vi "AddItemsToGraph.vi"(0 "GraphIn":refnum<class "Graph.lvclass">, 1 "graphics":refnum<class "Graphics.lvclass">, 2 "grid":refnum<class "Grid.lvclass">, 3 "ClassNodes":T5(array[cluster]) {"Point"."y" format="%.2f"; "Point"."x" format="%.2f"}, 4 "NoteNodes":T4(array[cluster]) {"Point"."y" format="%.2f"; "Point"."x" format="%.2f"}, 5 "error in (no error)":errorcluster, 7 "Links":T1[](array[typedef]), 9 "DoAContainCheck":bool, 11 "ClassNodesAtt/MethodIDs":cluster{string[], string[]}[](array[cluster]), 13 "NodeIndexiesToOnlyUpdate":i32[](array[numeric])) -> (14 "GraphOut":refnum<class "Graph.lvclass">, 16 "NodesCreated/Modified":refnum<class "AbstractNode.lvclass">[](array[class]), 19 "error out":errorcluster)   [LabVIEW 2020, in "Graph.lvclass"]
uses:
  <resource>/Framework/Providers/Open_GDS/UML/Graph_class/Graph.lvclass
  <resource>/Framework/Providers/Open_GDS/UML/Graphics_class/Graphics.lvclass
  <resource>/Framework/Providers/Open_GDS/UML/Grid_class/Grid.lvclass
  <resource>/Framework/Providers/Open_GDS/UML/General/Point/Point Point2D.ctl
  <resource>/Framework/Providers/Open_GDS/UML/Graph_class/AddItemsToGraph_Edges.ctl
  <resource>/Framework/Providers/Open_GDS/UML/DesignPattern/SubVIs/DesignPatterns_LinkType.ctl
  <resource>/Framework/Providers/Open_GDS/UML/AbstractNode_class/AbstractNode.lvclass
  <resource>/Framework/Providers/Open_GDS/UML/ClassNode_class/ClassNode.lvclass
  C:/Program Files (x86)/National Instruments/LabVIEW 2020/resource/Framework/Providers/Open_GDS/UML/AbstractNode_class/AbstractNode.lvclass
  <resource>/Framework/Providers/Open_GDS/UML/AbstractEdge_class/AbstractEdge.lvclass
  <resource>/Framework/Providers/Open_GDS/UML/ClassNode_class/ExternalSetTypes.ctl
  <resource>/Framework/Providers/Open_GDS/UML/MultiLineString_class/JustificationType.ctl
  <resource>/Framework/Providers/Open_GDS/UML/ClassRelationshipEdge_class/ExternaSetParamType.ctl
  <resource>/Framework/Providers/Open_GDS/UML/BentStyle_class/BentStyleType.ctl
  <resource>/Framework/Providers/Open_GDS/UML/ArrowHead_class/ArrowHeadType.ctl
  <resource>/Framework/Providers/Open_GDS/UML/LineStyle_class/LineStyleType.ctl
  <resource>/Framework/Providers/Open_GDS/UML/InterfaceNode_class/InterfaceNode.lvclass
  C:/Program Files (x86)/National Instruments/LabVIEW 2020/resource/Framework/Providers/Open_GDS/UML/ClassNode_class/ClassNode.lvclass
  <resource>/Framework/Providers/Open_GDS/UML/NoteNode_class/NoteNode.lvclass
  <resource>/Framework/Providers/Open_GDS/UML/ClassRelationshipEdge_class/ClassRelationshipEdge.lvclass
  C:/Program Files (x86)/National Instruments/LabVIEW 2020/resource/Framework/Providers/Open_GDS/UML/AbstractEdge_class/AbstractEdge.lvclass
  <resource>/Framework/Providers/Open_GDS/UML/NoteEdge_class/NoteEdge.lvclass
  <resource>/Framework/Providers/Open_GDS/UML/LineStyle_class/LineStyle.lvclass
  <resource>/Framework/Providers/Open_GDS/UML/MultiLineString_class/MultiLineString.lvclass
  <resource>/Framework/Providers/Open_GDS/UML/ArrowHead_class/ArrowHead.lvclass
  <resource>/Framework/Providers/Open_GDS/UML/BentStyle_class/BentStyle.lvclass
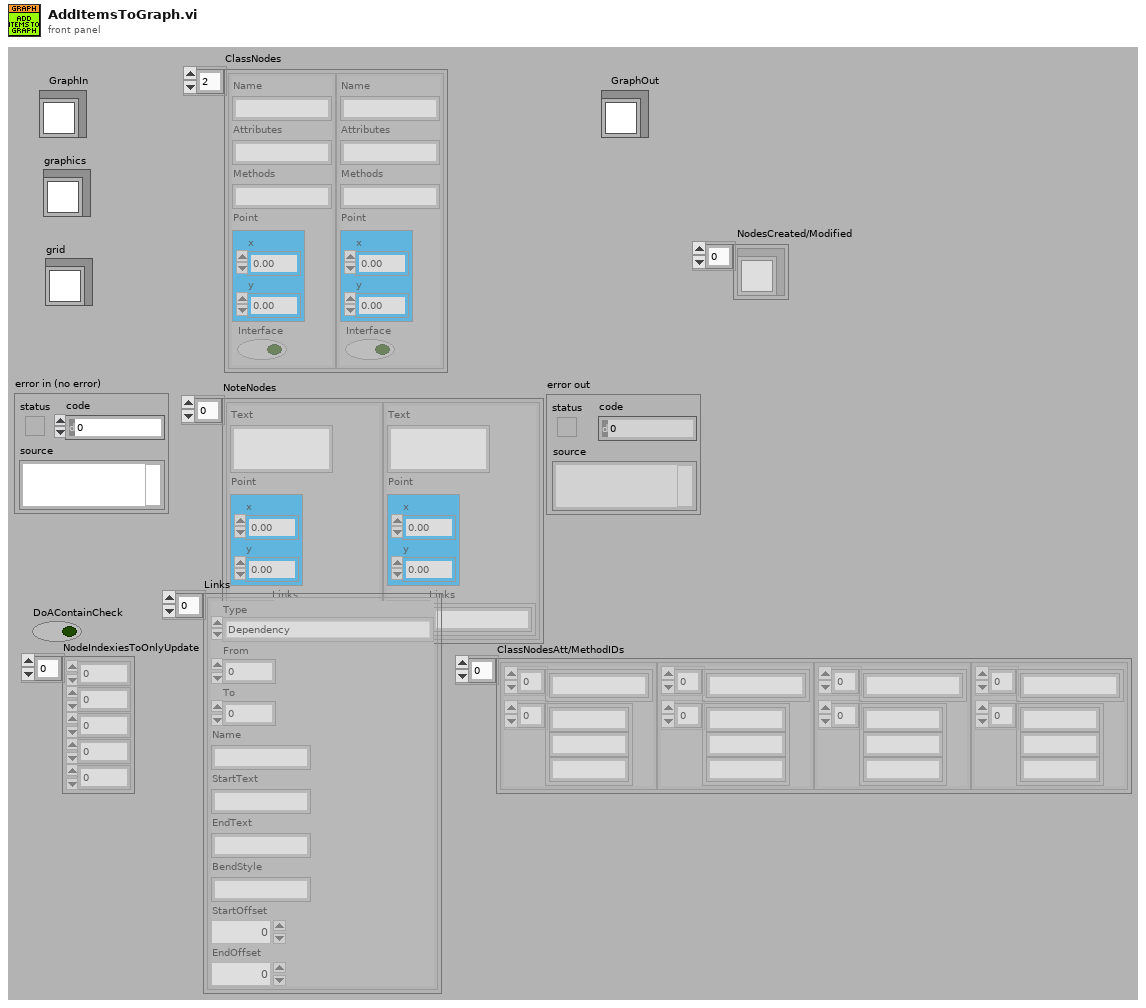
[diagram p1: front panel]
types:
  T1 = typedef "Graph.lvclass/AddItemsToGraph_Edges.ctl" = cluster{"Type":T2, "From":i32, "To":i32, "Name":string, "StartText":string, "EndText":string, "BendStyle":string, "StartOffset":i32, "EndOffset":i32}
  T2 = typedef "DesignPatterns_LinkType.ctl" = enum16{"Dependency", "Inheritance", "Interface", "Association", "Aggregation", "CompositeAggregation"}
  T3 = typedef "Point Point2D.ctl" = cluster{"x":dbl, "y":dbl}
  T4 = cluster{"Text":string, "Point":T3, "Links":string[]}[]
  T5 = cluster{"Name":string, "Attributes":string, "Methods":string, "Point":T3, "Interface":bool}[]
  T6 = cluster{"Text":string, "Cancelled":bool, "Classes":refnum<class "ClassNode.lvclass">[], "Edges":refnum<class "AbstractEdge.lvclass">[], "Notes":refnum<class "AbstractNode.lvclass">[], "NoteLinks":cluster{cluster{"reference out":refnum<class "ClassNode.lvclass">, "RightPoint":T3}[]}[], "ClassNodes":cluster{"Name":string, "Attributes":string, "Methods":string, "Point":T3, "Interface":bool}[], "Offset":T3, "nodes":refnum<class "AbstractNode.lvclass">[]}
  T7 = typedef "ClassNode.lvclass/ExternalSetTypes.ctl" = enum16{"Name", "Attributes", "Methods", "Position", "ShowMethods", "ShowAttributes", "ClassPath"}
  T8 = cluster{"reference out":refnum<class "ClassNode.lvclass">, "RightPoint":T3}[]
  T9 = typedef "MultiLineString.lvclass/JustificationType.ctl" = enum16{"LEFT", "CENTER", "RIGHT"}
  T10 = typedef "ClassRelationshipEdge.lvclass/ExternaSetParamType.ctl" = enum16{"StartLabel", "MidLabel", "EndLabel", "StartNode", "EndNode", "BendType", "StartArrow", "EndArrow", "StartOffset", "EndOffset"}
  T11 = typedef "BentStyle.lvclass/BentStyleType.ctl" = enum16{"STRAIGHT", "HV", "VH", "HVH", "VHV", "ARC"}
  T12 = typedef "ArrowHead.lvclass/ArrowHeadType.ctl" = enum16{"NONE", "TRIANGLE", "BLACK_TRIANGLE", "V", "HALF_V", "DIAMOND", "BLACK_DIAMOND"}
  T13 = typedef "LineStyle.lvclass/LineStyleType.ctl" = enum16{"SOLID", "DOTTED"}
  T14 = typedef "Rectangle Rectangle2D.ctl" = cluster{"x":dbl, "y":dbl, "width":dbl, "height":dbl}
  T15 = cluster{"Name":string, "Attributes":string, "Methods":string, "Point":T3, "Interface":bool}
  T16 = cluster{"reference out":refnum<class "ClassNode.lvclass">, "RightPoint":T3}
  T17 = cluster{"reference out":refnum<class "ClassNode.lvclass">, "UpperRightPoint":T3}
  T18 = cluster{"reference out":refnum<class "ClassNode.lvclass">, "UpperRightPoint":T3}[]
  T19 = cluster{cluster{"reference out":refnum<class "ClassNode.lvclass">, "RightPoint":T3}[]}
  T20 = cluster{cluster{"reference out":refnum<class "ClassNode.lvclass">, "RightPoint":T3}[]}[]
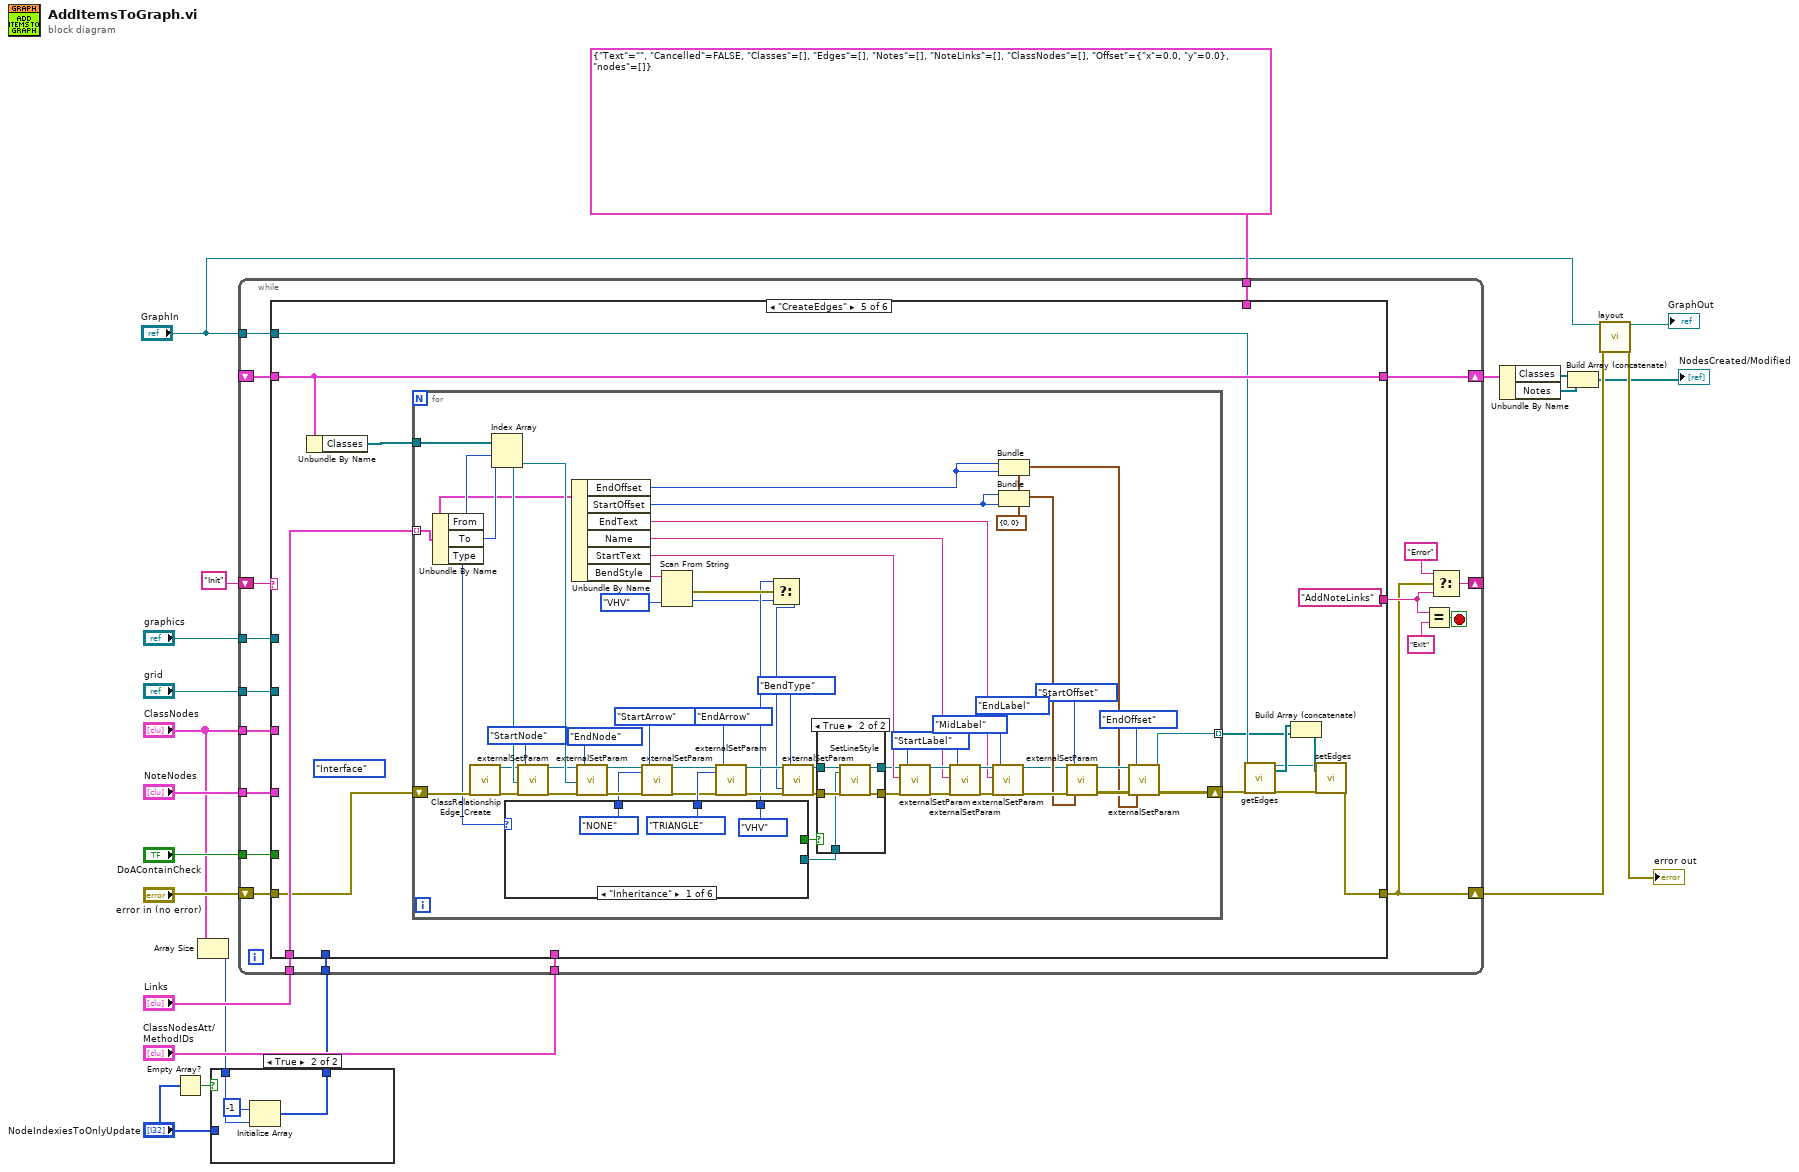
[diagram p0: block diagram]
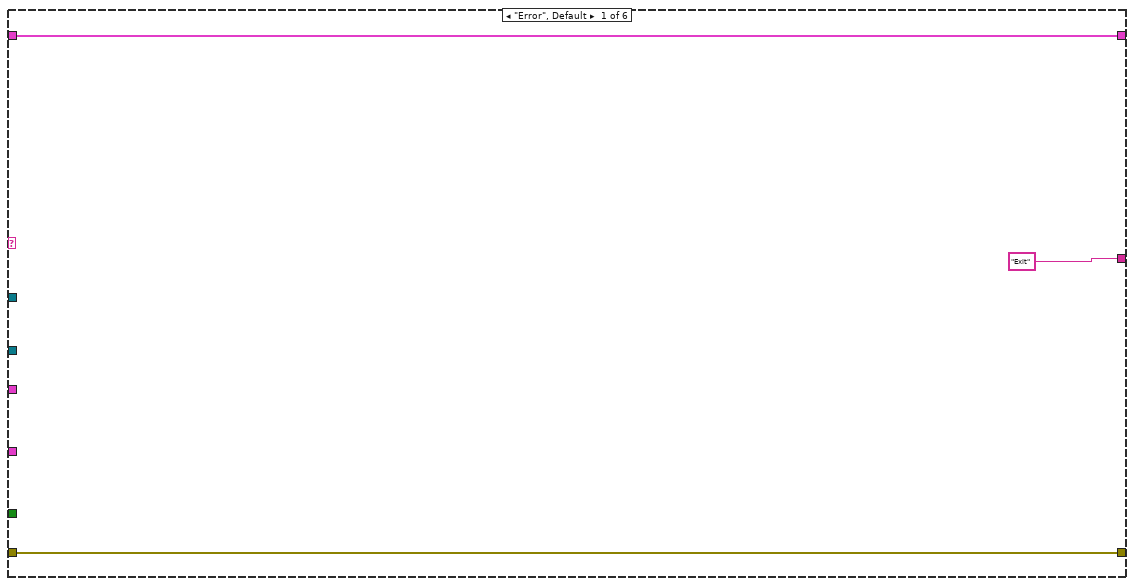
[diagram p3: hidden frame]
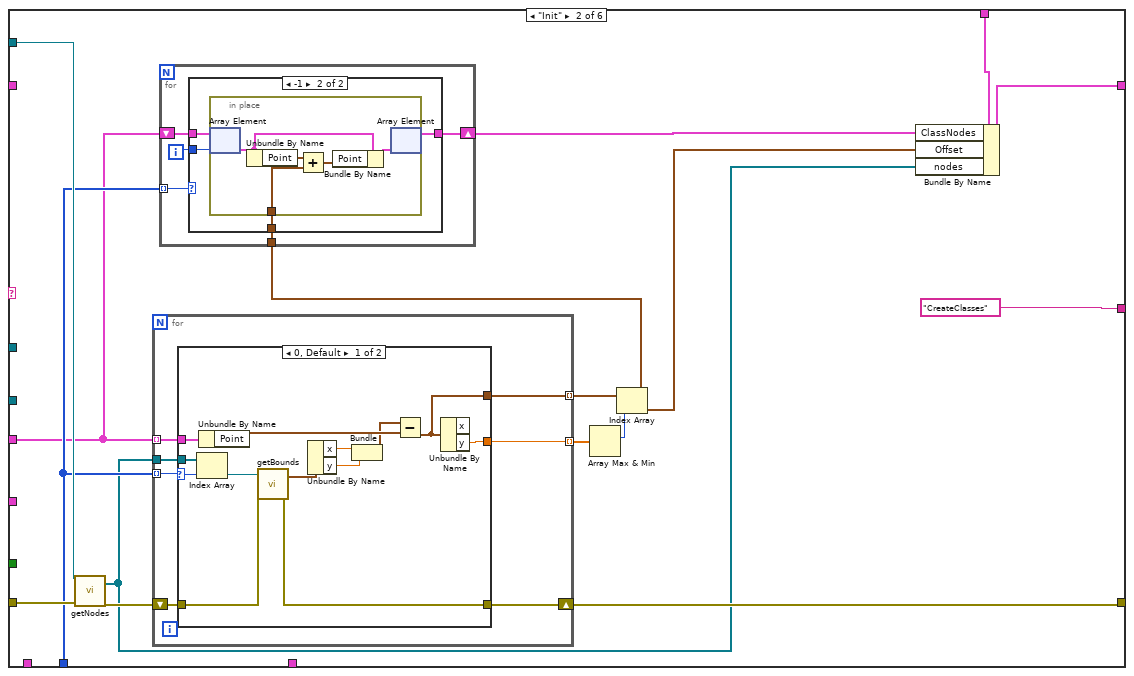
[diagram p4: hidden frame]
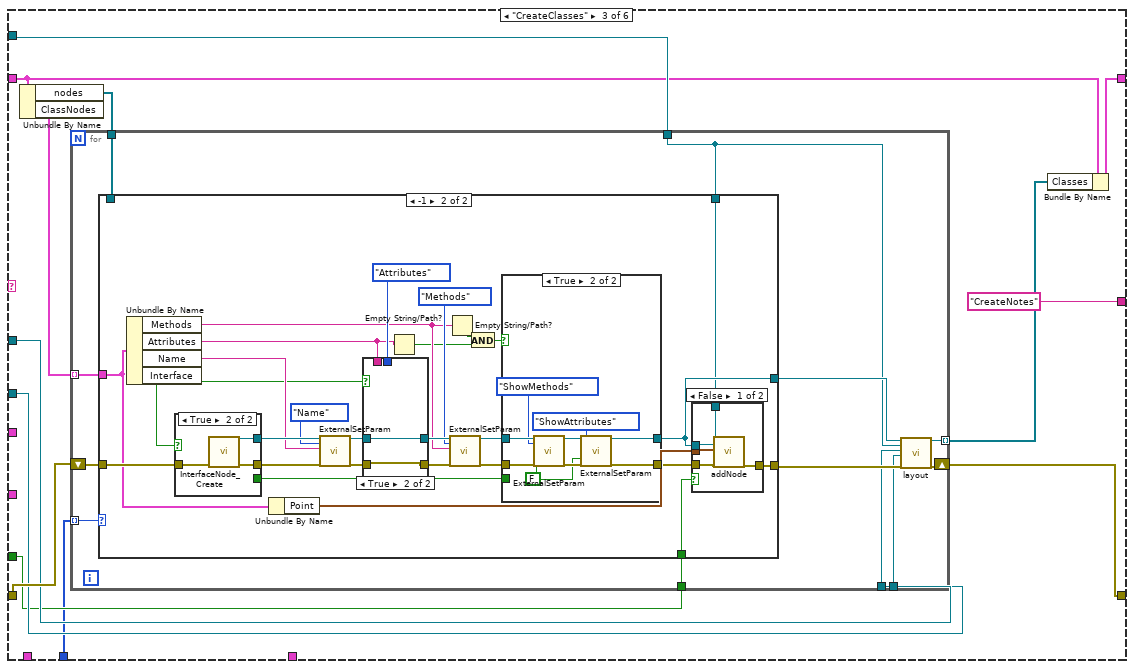
[diagram p7: hidden frame]
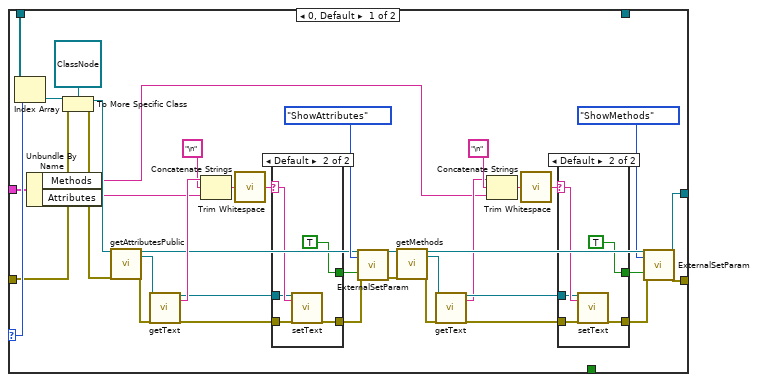
[diagram p8: hidden frame]
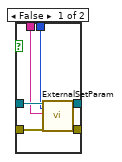
[diagram p11: hidden frame]
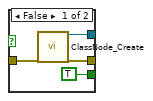
[diagram p12: hidden frame]
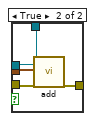
[diagram p14: hidden frame]
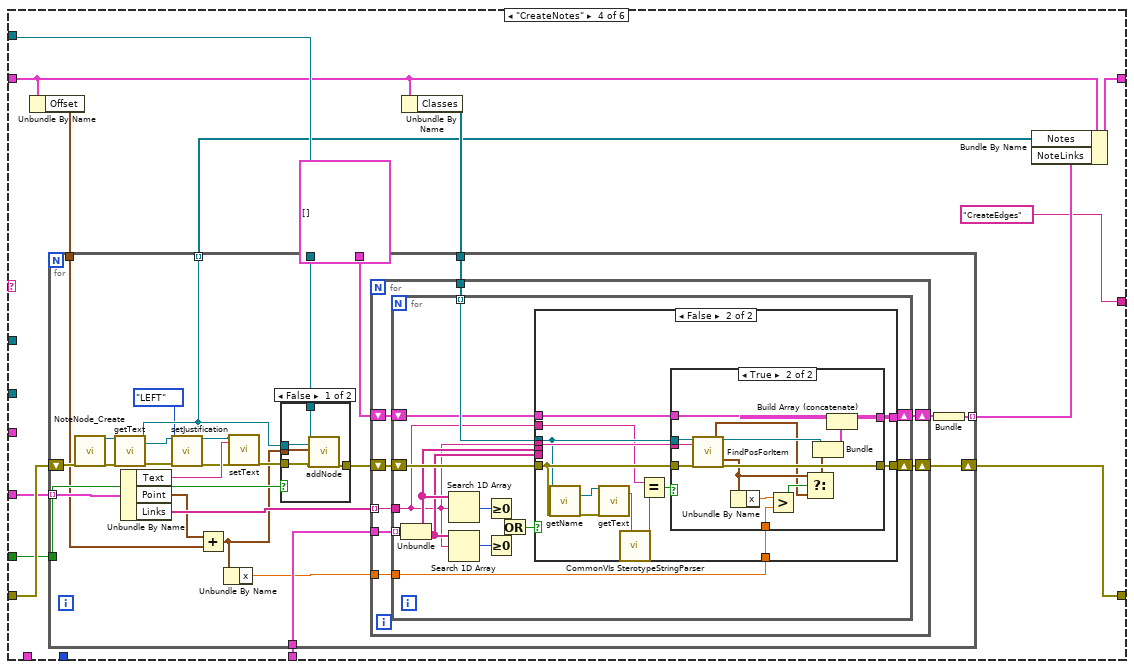
[diagram p15: hidden frame]
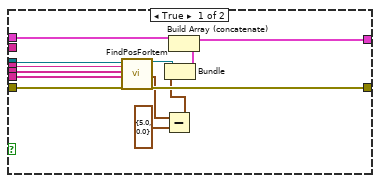
[diagram p16: hidden frame]
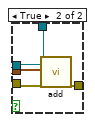
[diagram p18: hidden frame]
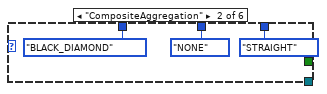
[diagram p20: hidden frame]
diagram:
  n1 = Empty Array?(array="NodeIndexiesToOnlyUpdate") -> (empty?=w8:bool)
  n2 = Array Size(array="ClassNodes") -> (size(s)=w5:i32)
  n3 = case shown="True" w8 {
    tunnel: "NodeIndexiesToOnlyUpdate" -> [w23 _]
    tunnel: w5 -> [_ w25]
    tunnel: [w23 w24] -> w4
    frame False {
    }
    frame True {
      n4 = Initialize Array(-1, w25) -> (w24:i32[])
    }
  }
  n5 = while {
    shift-right: [w39] -> w13
    shift-left: "error in (no error)" -> [w46]
    shift-right: [w44] -> _
    shift-left: "Init" -> [w45]
    shift-right: [w38] -> w22
    shift-left: _ -> [w37]
    tunnel: "GraphIn" -> [w36]
    tunnel: "graphics" -> [w35]
    tunnel: "grid" -> [w34]
    tunnel: T6 {"Text"="", "Cancelled"=FALSE, "Classes"=[], "Edges"=[], "Notes"=[], "NoteLinks"=[], "ClassNodes"=[], "Offset"={"x"=0.0, "y"=0.0}, "nodes"=[]} -> [w33]
    tunnel: "ClassNodes" -> [w27]
    tunnel: "NoteNodes" -> [w32]
    tunnel: "DoAContainCheck" -> [w31]
    tunnel: "Links" -> [w30]
    tunnel: "ClassNodesAtt/MethodIDs" -> [w29]
    tunnel: w4 -> [w28]
    stop <- w43 stop-if-true
    n6 = case shown="\"CreateEdges\"" w45 {
      tunnel: w46 -> [w49 w61 w111 w251 w363 w464]
      tunnel: [w49 w58 w110 w250 w362 w462] -> w39
      tunnel: ["Exit" "CreateClasses" "CreateNotes" "CreateEdges" "AddNoteLinks" "Exit"] -> w40
      tunnel: [w47 w63 w109 w245 w360 w458] -> w38
      tunnel: w37 -> [w47 _ w105 w242 w360 w459]
      tunnel: w36 -> [_ w60 w112 w252 w355 w463]
      tunnel: w35 -> [_ _ w107 _ _ _]
      tunnel: w34 -> [_ _ w106 _ _ _]
      tunnel: w33 -> [_ w62 _ _ _ _]
      tunnel: w32 -> [_ _ _ w249 _ _]
      tunnel: w31 -> [_ _ w103 w248 _ _]
      tunnel: w30 -> [_ _ _ _ w364 _]
      tunnel: w29 -> [_ _ _ w247 _ _]
      tunnel: w28 -> [_ w54 w102 _ _ _]
      tunnel: w27 -> [_ w52 _ _ _ _]
      frame "Error", Default {
      }
      frame "Init" {
        n7 = call-dynamic "getNodes.vi"("reference"=w60, "error in (no error)"=w61) -> ("nodes"=w50:refnum<class "AbstractNode.lvclass">[], "error out"=w59:errorcluster)  [unwired: 15 in, 1 out]
        n8 = for {
          tunnel: w50 -> [w86]
          tunnel: w54 -> [w83] mode=indexing
          shift-right: [w84] -> w58
          shift-left: w59 -> [w85]
          tunnel: w52 -> [w82] mode=indexing
          tunnel: [w81] -> w56 mode=indexing
          tunnel: [w80] -> w57 mode=indexing
          n9 = case shown="0, Default" w83 {
            selector: w83 -> [w95 _]
            tunnel: w86 -> [w99 _]
            tunnel: w85 -> [w97 w100]
            tunnel: [w96 w100] -> w84
            tunnel: w82 -> [w94 _]
            tunnel: [w88 _] -> w81
            tunnel: [w87 _] -> w80
            frame 0, Default {
              n10 = Index Array(array=w99, index=w95) -> (element=w98:refnum<class "AbstractNode.lvclass">)
              n11 = Unbundle By Name(w94) -> ("Point"=w90:T3)
              n12 = call-dynamic "getBounds.vi"("reference"=w98, "error in (no error)"=w97) -> ("bounds"=w93:T14, "error out"=w96:errorcluster)  [unwired: 15 in, 1 out]
              n13 = Unbundle By Name(w93) -> ("x"=w92:dbl, "y"=w91:dbl)
              n14 = Bundle("x"=w92, "y"=w91) -> (w89:cluster{"x":dbl, "y":dbl})  [unwired: 1 in]
              n15 = Subtract(x=w89, y=w90) -> (x-y=w88:T3)
              n16 = Unbundle By Name(w88) -> ("y"=w87:dbl)  [unwired: 1 out]
            }
            frame -1 {
            }
          }
        }
        n17 = Array Max & Min(array=w57) -> (max index (indices)=w55:i32)  [unwired: 3 out]
        n18 = Index Array(array=w56, index=w55) -> (element=w51:T3)
        n19 = for {
          tunnel: w54 -> [w69] mode=indexing
          tunnel: w51 -> [w67]
          shift-right: [w66] -> w53
          shift-left: w52 -> [w68]
          i -> [w65]
          n20 = case shown="-1" w69 {
            tunnel: w68 -> [w70 w73]
            tunnel: w67 -> [_ w74]
            tunnel: [w70 w72] -> w66
            tunnel: w65 -> [_ w71]
            frame 0, Default {
            }
            frame -1 {
              n21 = in-place {
                in-place-border: w74 -> [w77]
                n22 = in-place-array #1(w73, w71) -> (w76:T15)
                n23 = Unbundle By Name(w76) -> ("Point"=w79:T3)
                n24 = Add(x=w79, y=w77) -> (x+y=w78:T3)
                n25 = Bundle By Name(cluster=w76, "Point"=w78) -> (w75:T15)
                n26 = in-place-array #1(w75) -> (w72:T5)  [unwired: 1 out]
              }
            }
          }
        }
        n27 = Bundle By Name(cluster=w62, "ClassNodes"=w53, "Offset"=w51, "nodes"=w50) -> (w63:T6)
      }
      frame "CreateClasses" {
        n28 = Unbundle By Name(w105) -> ("nodes"=w101:refnum<class "AbstractNode.lvclass">[], "ClassNodes"=w104:T5)
        n29 = for {
          tunnel: w104 -> [w125] mode=indexing
          tunnel: w112 -> [w116]
          shift-right: [w121] -> w110
          shift-left: w111 -> [w124]
          tunnel: w103 -> [w123]
          tunnel: [w120] -> w108 mode=indexing
          tunnel: w107 -> [w119]
          tunnel: w106 -> [w118]
          tunnel: w102 -> [w114] mode=indexing
          tunnel: w101 -> [w115]
          n30 = case shown="-1" w114 {
            selector: w114 -> [w162 _]
            tunnel: w125 -> [w158 w178]
            tunnel: w124 -> [w160 w192]
            tunnel: w123 -> [_ w191]
            tunnel: [w127 w189] -> w122
            tunnel: [w126 w186] -> w117
            tunnel: w116 -> [_ w179]
            tunnel: w115 -> [w163 _]
            frame 0, Default {
              n31 = Index Array(array=w163, index=w162) -> (element=w161:refnum<class "AbstractNode.lvclass">)
              n32 = Unbundle By Name(w158) -> ("Methods"=w128:string, "Attributes"=w151:string)
              n33 = To More Specific Class(target class=refnum<class "ClassNode.lvclass"> refnum ("reference"), reference=w161, error in=w160) -> (specific class reference=w156:refnum<class "ClassNode.lvclass">, error out=w157:errorcluster)
              n34 = call <resource>:"getAttributesPublic.vi"("reference"=w156, "error in (no error)"=w157) -> ("reference out"=w144:refnum<class "ClassNode.lvclass">, "methods"=w154:refnum<class "MultiLineString.lvclass">, "error out"=w155:errorcluster)  [unwired: 15 in]
              n35 = call-dynamic "getText.vi"("reference"=w154, "error in (no error)"=w155) -> ("reference out"=w147:refnum<class "MultiLineString.lvclass">, "text"=w153:string, "error out"=w148:errorcluster)  [unwired: 15 in]
              n36 = Concatenate Strings(w153, "\n" ("string"), w151) -> (w150:string)
              n37 = call <vilib>:"Trim Whitespace.vi"("string"=w150) -> ("trimmed string"=w149:string)  [unwired: 1 in]
              n38 = case shown="Default" w149 {
                selector: w149 -> [_ w174]
                tunnel: w148 -> [w170 w175]
                tunnel: w147 -> [_ w173]
                tunnel: [w170 w172] -> w146
                tunnel: [_ TRUE] -> w143
                frame "" {
                }
                frame Default {
                  n39 = call-dynamic "setText.vi"("reference"=w173, "text"=w174, "error in (no error)"=w175) -> ("error out"=w172:errorcluster)  [unwired: 15 in, 1 out]
                }
              }
              n40 = call-dynamic "ExternalSetParam.vi"("reference"=w144, "setParameter"=ExternalSetTypes."ShowAttributes", "Boolean"=w143, "error in (no error)"=w146) -> ("reference out"=w130:refnum<class "ClassNode.lvclass">, "error out"=w129:errorcluster)  [unwired: 14 in]
              n41 = call <resource>:"getMethods.vi"("reference"=w130, "error in (no error)"=w129) -> ("reference out"=w141:refnum<class "ClassNode.lvclass">, "methods"=w132:refnum<class "MultiLineString.lvclass">, "error out"=w131:errorcluster)  [unwired: 15 in]
              n42 = call-dynamic "getText.vi"("reference"=w132, "error in (no error)"=w131) -> ("reference out"=w138:refnum<class "MultiLineString.lvclass">, "text"=w133:string, "error out"=w137:errorcluster)  [unwired: 15 in]
              n43 = Concatenate Strings(w133, "\n" ("string"), w128) -> (w135:string)
              n44 = call <vilib>:"Trim Whitespace.vi"("string"=w135) -> ("trimmed string"=w136:string)  [unwired: 1 in]
              n45 = case shown="Default" w136 {
                selector: w136 -> [_ w168]
                tunnel: w137 -> [w164 w169]
                tunnel: w138 -> [_ w167]
                tunnel: [w164 w166] -> w139
                tunnel: [_ TRUE] -> w142
                frame "" {
                }
                frame Default {
                  n46 = call-dynamic "setText.vi"("reference"=w167, "text"=w168, "error in (no error)"=w169) -> ("error out"=w166:errorcluster)  [unwired: 15 in, 1 out]
                }
              }
              n47 = call-dynamic "ExternalSetParam.vi"("reference"=w141, "setParameter"=ExternalSetTypes."ShowMethods", "Boolean"=w142, "error in (no error)"=w139) -> ("reference out"=w126:refnum<class "ClassNode.lvclass">, "error out"=w127:errorcluster)  [unwired: 14 in]
            }
            frame -1 {
              n48 = Unbundle By Name(w178) -> ("Methods"=w184:string, "Attributes"=w183:string, "Name"=w193:string, "Interface"=w177:bool)
              n49 = case shown="True" w177 {
                tunnel: [w214 w215] -> w202
                tunnel: [w213 w217] -> w201
                tunnel: w192 -> [w212 w216]
                tunnel: [TRUE ("Boolean") _] -> w176
                frame False {
                  n50 = call <resource>:"ClassNode_Create.vi"("error in (no error)"=w212) -> ("reference out"=w214:refnum<class "ClassNode.lvclass">, "error out"=w213:errorcluster)  [unwired: 1 in, 16 out]
                }
                frame True {
                  n51 = call <resource>:"InterfaceNode_Create.vi"("error in (no error)"=w216) -> ("reference out"=w215:refnum<class "InterfaceNode.lvclass">, "error out"=w217:errorcluster)  [unwired: 17 in]
                }
              }
              n52 = Unbundle By Name(w178) -> ("Point"=w190:T3)
              n53 = call-dynamic "ExternalSetParam.vi"("reference"=w202, "setParameter"=ExternalSetTypes."Name", "string"=w193, "error in (no error)"=w201) -> ("reference out"=w199:refnum<class "ClassNode.lvclass">, "error out"=w198:errorcluster)  [unwired: 14 in]
              n54 = case shown="True" w177 {
                tunnel: w199 -> [w208 w210]
                tunnel: w198 -> [w207 w209]
                tunnel: ExternalSetTypes."Attributes" ("setParameter") -> [w206 _]
                tunnel: [w205 w209] -> w196
                tunnel: [w204 w210] -> w195
                tunnel: w183 -> [w203 _]
                frame False {
                  n55 = call-dynamic "ExternalSetParam.vi"("reference"=w208, "setParameter"=w206, "string"=w203, "error in (no error)"=w207) -> ("reference out"=w204:refnum<class "ClassNode.lvclass">, "error out"=w205:errorcluster)  [unwired: 14 in]
                }
                frame True {
                }
              }
              n56 = Empty String/Path?(string/path=w183) -> (empty?=w181:bool)
              n57 = Empty String/Path?(string/path=w184) -> (empty?=w182:bool)
              n58 = call-dynamic "ExternalSetParam.vi"("reference"=w195, "setParameter"=ExternalSetTypes."Methods", "string"=w184, "error in (no error)"=w196) -> ("reference out"=w185:refnum<class "ClassNode.lvclass">, "error out"=w188:errorcluster)  [unwired: 14 in]
              n59 = And(x=w182, y=w181) -> (x .and. y?=w180:bool)
              n60 = case shown="True" w180 {
                tunnel: w188 -> [w218 w228]
                tunnel: [w218 w226] -> w187
                tunnel: [w219 w225] -> w186
                tunnel: w185 -> [w219 w223]
                tunnel: w176 -> [_ _]
                frame False {
                }
                frame True {
                  w220 = FALSE ("Boolean")
                  n61 = call-dynamic "ExternalSetParam.vi"("reference"=w223, "setParameter"=ExternalSetTypes."ShowMethods", "Boolean"=w220, "error in (no error)"=w228) -> ("reference out"=w224:refnum<class "ClassNode.lvclass">, "error out"=w227:errorcluster)  [unwired: 14 in]
                  n62 = call-dynamic "ExternalSetParam.vi"("reference"=w224, "setParameter"=ExternalSetTypes."ShowAttributes", "Boolean"=w220, "error in (no error)"=w227) -> ("reference out"=w225:refnum<class "ClassNode.lvclass">, "error out"=w226:errorcluster)  [unwired: 14 in]
                }
              }
              n63 = case shown="False" w191 {
                tunnel: w179 -> [w232 w238]
                tunnel: w190 -> [w233 w237]
                tunnel: [w229 w236] -> w189
                tunnel: w186 -> [w231 w235]
                tunnel: w187 -> [w230 w234]
                frame False {
                  n64 = call-dynamic "addNode.vi"("reference"=w232, "node"=w231, "point"=w233, "error in (no error)"=w230) -> ("error out"=w229:errorcluster)  [unwired: 14 in, 1 out]
                }
                frame True {
                  n65 = call-dynamic "add.vi"("reference"=w238, "node"=w235, "point"=w237, "error in (no error)"=w234) -> ("error out"=w236:errorcluster)  [unwired: 13 in, 2 out]
                }
              }
            }
          }
          n66 = call-dynamic "layout.vi"("reference"=w117, "graph"=w116, "graphics"=w119, "grid"=w118, "error in (no error)"=w122) -> ("reference out"=w120:refnum<class "ClassNode.lvclass">, "error out"=w121:errorcluster)  [unwired: 13 in]
        }
        n67 = Bundle By Name(cluster=w105, "Classes"=w108) -> (w109:T6)
      }
      frame "CreateNotes" {
        n68 = Unbundle By Name(w242) -> ("Offset"=w241:T3)
        n69 = Unbundle By Name(w242) -> ("Classes"=w246:refnum<class "ClassNode.lvclass">[])
        n70 = for {
          tunnel: w252 -> [w277]
          shift-right: [w269] -> w250
          shift-left: w251 -> [w276]
          tunnel: w249 -> [w272] mode=indexing
          tunnel: w248 -> [w270]
          tunnel: w247 -> [w266]
          tunnel: w246 -> [w267]
          tunnel: [w264] -> w244 mode=indexing
          tunnel: [w263] -> w243 mode=indexing
          tunnel: w241 -> [w257]
          tunnel: T8 [] -> [w255]
          n71 = call <resource>:"NoteNode_Create.vi"("error in (no error)"=w276) -> ("reference out"=w275:refnum<class "NoteNode.lvclass">, "error out"=w274:errorcluster)  [unwired: 17 in]
          n72 = call-dynamic "getText.vi"("reference"=w275, "error in (no error)"=w274) -> ("reference out"=w263:refnum<class "NoteNode.lvclass">, "text"=w262:refnum<class "MultiLineString.lvclass">, "error out"=w261:errorcluster)  [unwired: 15 in]
          n73 = Unbundle By Name(w272) -> ("Text"=w271:string, "Point"=w256:T3, "Links"=w268:string[])
          n74 = call <resource>:"setJustification.vi"("reference"=w262, "justification"=JustificationType."LEFT", "error in (no error)"=w261) -> ("reference out"=w259:refnum<class "MultiLineString.lvclass">, "error out"=w260:errorcluster)  [unwired: 15 in]
          n75 = Add(x=w256, y=w257) -> (x+y=w254:T3)
          n76 = Unbundle By Name(w254) -> ("x"=w253:dbl)
          n77 = call-dynamic "setText.vi"("reference"=w259, "text"=w271, "error in (no error)"=w260) -> ("error out"=w273:errorcluster)  [unwired: 15 in, 1 out]
          n78 = case shown="False" w270 {
            tunnel: w277 -> [w346 w352]
            tunnel: w254 -> [w347 w351]
            tunnel: [w343 w350] -> w269
            tunnel: w263 -> [w345 w349]
            tunnel: w273 -> [w344 w348]
            frame False {
              n79 = call-dynamic "addNode.vi"("reference"=w346, "node"=w345, "point"=w347, "error in (no error)"=w344) -> ("error out"=w343:errorcluster)  [unwired: 14 in, 1 out]
            }
            frame True {
              n80 = call-dynamic "add.vi"("reference"=w352, "node"=w349, "point"=w351, "error in (no error)"=w348) -> ("error out"=w350:errorcluster)  [unwired: 13 in, 2 out]
            }
          }
          n81 = for {
            shift-right: [w284] -> _
            shift-left: w269 -> [w285]
            tunnel: w268 -> [w282] mode=indexing
            tunnel: w267 -> [w283]
            tunnel: w266 -> [w281]
            shift-right: [w279] -> w265
            shift-left: w255 -> [w280]
            tunnel: w253 -> [w278]
            n82 = for {
              shift-right: [w299] -> w284
              shift-left: w285 -> [w300]
              tunnel: w283 -> [w298] mode=indexing
              tunnel: w281 -> [w297] mode=indexing
              tunnel: w282 -> [w287]
              shift-right: [w288] -> w279
              shift-left: w280 -> [w289]
              tunnel: w278 -> [w286]
              n83 = Unbundle(w297) -> (w292:string[], w291:string[])
              n84 = Search 1D Array(1D array=w292, element=w287) -> (index of element=w296:i32)  [unwired: 1 in]
              n85 = Search 1D Array(1D array=w291, element=w287) -> (index of element=w295:i32)  [unwired: 1 in]
              n86 = Greater Or Equal To 0?(x=w296) -> (x >= 0?=w294:bool)
              n87 = Greater Or Equal To 0?(x=w295) -> (x >= 0?=w293:bool)
              n88 = Or(x=w294, y=w293) -> (x .or. y?=w290:bool)
              n89 = case shown="False" w290 {
                tunnel: w300 -> [w313 w320]
                tunnel: [w312 w326] -> w299
                tunnel: w298 -> [w311 w319]
                tunnel: w287 -> [w310 w325]
                tunnel: w292 -> [w309 _]
                tunnel: w291 -> [w308 _]
                tunnel: w289 -> [w307 w324]
                tunnel: [w306 w323] -> w288
                tunnel: w287 -> [_ w318]
                tunnel: w286 -> [_ w314]
                frame True {
                  n90 = call-dynamic "FindPosForItem.vi"("reference"=w311, "SearchItem"=w310, "AttributesIDs"=w309, "MethodIDs"=w308, "error in (no error)"=w313) -> ("reference out"=w305:refnum<class "ClassNode.lvclass">, "RightPoint"=w303:T3, "error out"=w312:errorcluster)  [unwired: 8 in, 4 out]
                  n91 = Subtract(x=w303, y=T3 {"x"=5.0, "y"=0.0}) -> (x-y=w301:T3)
                  n92 = Bundle("reference out"=w305, "RightPoint"=w301) -> (w304:T16)  [unwired: 1 in]
                  n93 = Build Array (concatenate)(w307, w304) -> (w306:T8)
                }
                frame False {
                  n94 = call-dynamic "getName.vi"("reference"=w319, "error in (no error)"=w320) -> ("name"=w321:refnum<class "MultiLineString.lvclass">, "error out"=w322:errorcluster)  [unwired: 15 in, 1 out]
                  n95 = call-dynamic "getText.vi"("reference"=w321, "error in (no error)"=w322) -> ("text"=w316:string)  [unwired: 15 in, 2 out]
                  n96 = call <resource>:"CommonVIs SterotypeStringParser.vi"("SterotypeStringIn"=w316) -> ("Name"=w315:string)  [unwired: 15 in, 3 out]
                  n97 = Equal?(x=w318, y=w315) -> (x = y?=w317:bool)
                  n98 = case shown="True" w317 {
                    tunnel: [w328 w342] -> w326
                    tunnel: w325 -> [_ w341]
                    tunnel: w324 -> [w327 w340]
                    tunnel: [w327 w337] -> w323
                    tunnel: w320 -> [w328 w336]
                    tunnel: w319 -> [_ w335]
                    tunnel: w314 -> [_ w333]
                    frame False {
                    }
                    frame True {
                      n99 = call-dynamic "FindPosForItem.vi"("reference"=w335, "SearchItem"=w341, "error in (no error)"=w336) -> ("UpperRightPoint"=w330:T3, "reference out"=w339:refnum<class "ClassNode.lvclass">, "UpperLeftPoint"=w331:T3, "error out"=w342:errorcluster)  [unwired: 10 in, 3 out]
                      n100 = Unbundle By Name(w331) -> ("x"=w334:dbl)
                      n101 = Greater?(x=w334, y=w333) -> (0:w332:bool)
                      n102 = Select(t=w331, s=w332, f=w330) -> (s? t:f=w329:T3)
                      n103 = Bundle("reference out"=w339, "UpperRightPoint"=w329) -> (w338:T17)  [unwired: 1 in]
                      n104 = Build Array (concatenate)(w340, w338) -> (w337:T18)
                    }
                  }
                }
              }
            }
          }
          n105 = Bundle(w265) -> (w264:T19)  [unwired: 1 in]
        }
        n106 = Bundle By Name(cluster=w242, "Notes"=w243, "NoteLinks"=w244) -> (w245:T6)
      }
      frame "CreateEdges" {
        (unwired) DesignPatterns_LinkType."Interface" ("Type")
        n107 = Unbundle By Name(w360) -> ("Classes"=w365:refnum<class "ClassNode.lvclass">[])
        n108 = for {
          shift-right: [w366] -> w359
          shift-left: w363 -> [w422]
          tunnel: w365 -> [w425]
          tunnel: w364 -> [w418] mode=indexing
          tunnel: [w369] -> w353 mode=indexing
          w374 = cluster{"x":i32, "y":i32} {"x"=0, "y"=0} ("ConnectionOffset")
          n109 = Unbundle By Name(w418) -> ("From"=w424:i32, "To"=w423:i32, "Type"=w392:T2)
          n110 = call <resource>:"ClassRelationshipEdge_Create.vi"("error in (no error)"=w422) -> ("reference out"=w398:refnum<class "ClassRelationshipEdge.lvclass">, "error out"=w399:errorcluster)  [unwired: 1 in, 16 out]
          n111 = Index Array(array=w425, index #1=w424, index #2=w423) -> (element #1=w421:refnum<class "ClassNode.lvclass">, element #2=w420:refnum<class "ClassNode.lvclass">)
          n112 = case shown="\"Inheritance\"" w392 {
            tunnel: [BentStyleType."VHV" ("bentStyle") BentStyleType."STRAIGHT" ("bentStyle") BentStyleType."STRAIGHT" ("bentStyle") BentStyleType."HVH" ("bentStyle") BentStyleType."HVH" ("bentStyle") BentStyleType."VHV" ("bentStyle")] -> w381
            tunnel: [ArrowHeadType."TRIANGLE" ("arrowHead") ArrowHeadType."NONE" ("arrowHead") ArrowHeadType."NONE" ("arrowHead") ArrowHeadType."V" ("arrowHead") ArrowHeadType."V" ("arrowHead") ArrowHeadType."TRIANGLE" ("arrowHead")] -> w405
            tunnel: [ArrowHeadType."NONE" ("arrowHead") ArrowHeadType."BLACK_DIAMOND" ("arrowHead") ArrowHeadType."DIAMOND" ("arrowHead") ArrowHeadType."NONE" ("arrowHead") ArrowHeadType."NONE" ("arrowHead") ArrowHeadType."NONE" ("arrowHead")] -> w391
            tunnel: [_ _ _ _ TRUE TRUE] -> w386
            tunnel: [_ _ _ _ w445 w451] -> w385
            frame "Inheritance" {
            }
            frame "CompositeAggregation" {
            }
            frame "Aggregation" {
            }
            frame "Association", Default {
            }
            frame "Dependency" {
              n113 = call <resource>:"getObject.vi"("lineStyle"=LineStyleType."DOTTED") -> ("reference out"=w445:refnum<class "LineStyle.lvclass">)  [unwired: 1 in, 17 out]
            }
            frame "Interface" {
              n114 = call <resource>:"getObject.vi"("lineStyle"=LineStyleType."DOTTED") -> ("reference out"=w451:refnum<class "LineStyle.lvclass">)  [unwired: 1 in, 17 out]
            }
          }
          n115 = call-dynamic "externalSetParam.vi"("reference"=w398, "node"=w421, "error in (no error)"=w399, "setParam"=ExternaSetParamType."StartNode") -> ("reference out"=w401:refnum<class "ClassRelationshipEdge.lvclass">, "error out"=w402:errorcluster)  [unwired: 14 in]
          n116 = Unbundle By Name(w418) -> ("EndOffset"=w373:i32, "StartOffset"=w376:i32, "EndText"=w410:string, "Name"=w413:string, "StartText"=w417:string, "BendStyle"=w384:string)
          n117 = call-dynamic "externalSetParam.vi"("reference"=w401, "node"=w420, "error in (no error)"=w402, "setParam"=ExternaSetParamType."EndNode") -> ("reference out"=w397:refnum<class "ClassRelationshipEdge.lvclass">, "error out"=w396:errorcluster)  [unwired: 14 in]
          n118 = call-dynamic "externalSetParam.vi"("reference"=w397, "arrowHead"=w391, "error in (no error)"=w396, "setParam"=ExternaSetParamType."StartArrow") -> ("reference out"=w395:refnum<class "ClassRelationshipEdge.lvclass">, "error out"=w394:errorcluster)  [unwired: 14 in]
          n119 = Scan From String(input string=w384, default 1=BentStyleType."VHV" ("bentStyle")) -> (error out=w382:errorcluster, output 1=w380:T11)  [unwired: 3 in, 2 out]
          n120 = call-dynamic "externalSetParam.vi"("reference"=w395, "arrowHead"=w405, "error in (no error)"=w394, "setParam"=ExternaSetParamType."EndArrow") -> ("reference out"=w406:refnum<class "ClassRelationshipEdge.lvclass">, "error out"=w407:errorcluster)  [unwired: 14 in]
          n121 = Select(t=w381, s=w382, f=w380) -> (s? t:f=w379:T11)
          n122 = call-dynamic "externalSetParam.vi"("reference"=w406, "bentStyle"=w379, "error in (no error)"=w407, "setParam"=ExternaSetParamType."BendType") -> ("reference out"=w389:refnum<class "ClassRelationshipEdge.lvclass">, "error out"=w388:errorcluster)  [unwired: 14 in]
          n123 = case shown="True" w386 {
            tunnel: [w427 w432] -> w390
            tunnel: w389 -> [w426 w431]
            tunnel: w388 -> [w427 w430]
            tunnel: [w426 w429] -> w387
            tunnel: w385 -> [_ w428]
            frame False {
            }
            frame True {
              n124 = call-dynamic "SetLineStyle.vi"("reference"=w431, "lineStyle"=w428, "error in (no error)"=w430) -> ("reference out"=w429:refnum<class "ClassRelationshipEdge.lvclass">, "error out"=w432:errorcluster)  [unwired: 15 in]
            }
          }
          n125 = call-dynamic "externalSetParam.vi"("reference"=w387, "string"=w417, "error in (no error)"=w390, "setParam"=ExternaSetParamType."StartLabel") -> ("reference out"=w414:refnum<class "ClassRelationshipEdge.lvclass">, "error out"=w415:errorcluster)  [unwired: 14 in]
          n126 = call-dynamic "externalSetParam.vi"("reference"=w414, "string"=w413, "error in (no error)"=w415, "setParam"=ExternaSetParamType."MidLabel") -> ("reference out"=w411:refnum<class "ClassRelationshipEdge.lvclass">, "error out"=w412:errorcluster)  [unwired: 14 in]
          n127 = call-dynamic "externalSetParam.vi"("reference"=w411, "string"=w410, "error in (no error)"=w412, "setParam"=ExternaSetParamType."EndLabel") -> ("reference out"=w370:refnum<class "ClassRelationshipEdge.lvclass">, "error out"=w378:errorcluster)  [unwired: 14 in]
          n128 = Bundle(cluster=w374, "x"=w373, "y"=w373) -> (w367:cluster{"x":i32, "y":i32})
          n129 = Bundle(cluster=w374, "x"=w376, "y"=w376) -> (w375:cluster{"x":i32, "y":i32})
          n130 = call-dynamic "externalSetParam.vi"("reference"=w370, "error in (no error)"=w378, "setParam"=ExternaSetParamType."StartOffset", "ConnectionOffset"=w375) -> ("reference out"=w371:refnum<class "ClassRelationshipEdge.lvclass">, "error out"=w372:errorcluster)  [unwired: 14 in]
          n131 = call-dynamic "externalSetParam.vi"("reference"=w371, "error in (no error)"=w372, "setParam"=ExternaSetParamType."EndOffset", "ConnectionOffset"=w367) -> ("reference out"=w369:refnum<class "ClassRelationshipEdge.lvclass">, "error out"=w366:errorcluster)  [unwired: 14 in]
        }
        n132 = call-dynamic "getEdges.vi"("reference"=w355, "error in (no error)"=w359) -> ("reference out"=w354:refnum<class "Graph.lvclass">, "edges"=w357:refnum<class "AbstractEdge.lvclass">[], "error out"=w358:errorcluster)  [unwired: 15 in]
        n133 = Build Array (concatenate)(w357, w353) -> (w356:refnum<class "AbstractEdge.lvclass">[])
        n134 = call-dynamic "setEdges.vi"("reference"=w354, "edges"=w356, "error in (no error)"=w358) -> ("error out"=w362:errorcluster)  [unwired: 15 in, 1 out]
      }
      frame "AddNoteLinks" {
        n135 = Unbundle By Name(w459) -> ("Notes"=w460:refnum<class "AbstractNode.lvclass">[], "NoteLinks"=w465:T20)
        n136 = for {
          tunnel: w465 -> [w472] mode=indexing
          tunnel: w460 -> [w473] mode=indexing
          shift-right: [w468] -> w462
          shift-left: w464 -> [w470]
          tunnel: w463 -> [w469]
          shift-right: [w466] -> w457
          shift-left: w460 -> [w467]
          n137 = Unbundle(w472) -> (w471:T8)
          n138 = for {
            tunnel: w473 -> [w494]
            tunnel: w471 -> [w485] mode=indexing
            shift-right: [w484] -> w468
            shift-left: w470 -> [w481]
            tunnel: w469 -> [w495]
            shift-right: [w475] -> w466
            shift-left: w467 -> [w476]
            n139 = Unbundle(w485) -> ("reference out"=w480:refnum<class "ClassNode.lvclass">, "RightPoint"=w483:T3)
            n140 = Unbundle(w483) -> ()  [unwired: 2 out]
            n141 = call-dynamic "getBounds.vi"("reference"=w494, "error in (no error)"=w481) -> ("bounds"=w493:T14, "error out"=w487:errorcluster)  [unwired: 15 in, 1 out]
            n142 = Unbundle(w493) -> ("x"=w492:dbl, "y"=w491:dbl)  [unwired: 2 out]
            n143 = call <resource>:"NoteEdge_Create.vi"("error in (no error)"=w487) -> ("reference out"=w477:refnum<class "NoteEdge.lvclass">, "error out"=w486:errorcluster)  [unwired: 17 in]
            n144 = Increment(x=w492) -> (x+1=w488:dbl)
            n145 = Increment(x=w491) -> (x+1=w489:dbl)
            n146 = Bundle(cluster=T3 {"x"=0.0, "y"=0.0}, "x"=w488, "y"=w489) -> (w482:T3)
            n147 = call-dynamic "connect.vi"("reference"=w495, "egde"=w477, "p1"=w482, "p2"=w483, "error in (no error)"=w486) -> ("error out"=w479:errorcluster)  [unwired: 12 in, 2 out]
            n148 = call-dynamic "getEnd.vi"("reference"=w477, "error in (no error)"=w479) -> ("endNode"=w474:refnum<class "AbstractNode.lvclass">, "error out"=w478:errorcluster)  [unwired: 14 in, 2 out]
            n149 = call-dynamic "addChild.vi"("reference"=w480, "node"=w474, "error in (no error)"=w478) -> ("error out"=w484:errorcluster)  [unwired: 15 in, 1 out]
            n150 = Build Array (concatenate)(w476, w474) -> (w475:refnum<class "AbstractNode.lvclass">[])
          }
        }
        n151 = Bundle By Name(cluster=w459, "Notes"=w457) -> (w458:T6)
      }
    }
    n152 = Equal?(x=w40, y="Exit") -> (x = y?=w43:bool)
    n153 = Select(t="Error", s=w39, f=w40) -> (s? t:f=w44:string)
  }
  n154 = Unbundle By Name(w22) -> ("Classes"=w3:refnum<class "ClassNode.lvclass">[], "Notes"=w2:refnum<class "AbstractNode.lvclass">[])
  n155 = Build Array (concatenate)(w3, w2) -> (→"NodesCreated/Modified":refnum<class "AbstractNode.lvclass">[])
  n156 = call-dynamic "layout.vi"("reference"="GraphIn", "error in (no error)"=w13) -> ("reference out"=→"GraphOut":refnum<class "Graph.lvclass">, "error out"=→"error out":errorcluster)  [unwired: 16 in]
